vi "Read Door Buttons.vi"(8 "error in (no error)":errorcluster, 11 "Abstract User Console in":refnum<class "Abstract User Console.lvclass">) -> (0 "error out":errorcluster, 2 "Door Buttons":T1, 3 "Abstract User Console out":refnum<class "Abstract User Console.lvclass">)   [LabVIEW 2019, in "Abstract User Console Actor.lvlib" / "Abstract User Console.lvclass"]
uses:
  Abstract User Console.lvclass
  User Console Actor/User Console/Door Buttons.ctl
  User Console Actor/User Console/User Console.lvclass
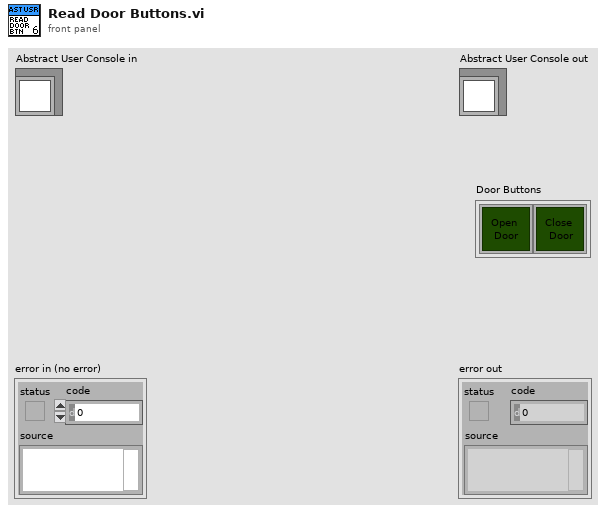
[diagram p1: front panel]
types:
  T1 = typedef "User Console Actor.lvlib/User Console.lvclass/Door Buttons.ctl" = cluster{"Open Door":bool, "Close Door":bool}
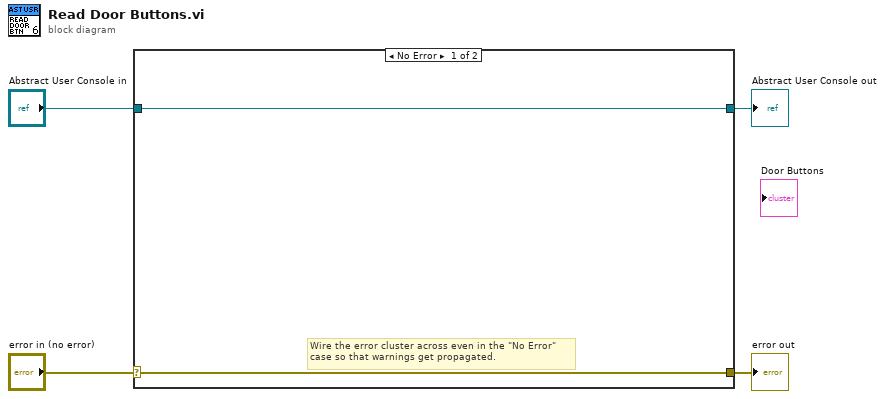
[diagram p0: block diagram]
diagram:
  n1 = case shown="No Error" "error in (no error)" {
    selector: "error in (no error)" -> [w5 w8]
    tunnel: [w5 w8] -> w3
    tunnel: [w6 w7] -> w1
    tunnel: "Abstract User Console in" -> [w6 w7]
    frame No Error {
      # "Wire the error cluster across even in the \"No Error\"\ncase so that warnings get propagated."
    }
    frame Error {
    }
  }
  "error out" <- w3
  "Abstract User Console out" <- w1
